vi "SetScale.vi"(10 "Scale":refnum<class "Scale_PiecedLinear.lvclass">, 11 "Sig_AI in":refnum<class "AO.lvclass">) -> (3 "Sig_AI out":refnum<class "AO.lvclass">)   [LabVIEW 2019]
uses:
  AO.lvclass
  D:/GIT H4000/H4000/src/Signal_class/Signal.lvclass
  D:/GIT H4000/H4000/src/Proccess_class/Proccess.lvclass
  PiecedLinearScale_class/Scale_PiecedLinear.lvclass
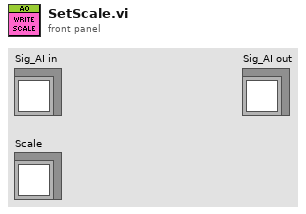
[diagram p1: front panel]
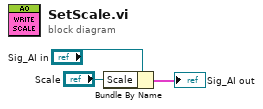
[diagram p0: block diagram]
diagram:
  n1 = Bundle By Name(cluster="Sig_AI in", "Scale"="Scale") -> (→"Sig_AI out":cluster{})
